vi "SUBVI_Image_to_Binary.vi"(11 "Image-in":T1) -> (0 "Red Binary":string[][](array[string]), 1 "Red Number":u8[][](array[numeric]), 2 "Blue Number":u8[][](array[numeric]), 3 "image_width":i32, 4 "Green Number":u8[][](array[numeric]), 5 "image_length":i32, 6 "Green Binary":string[][](array[string]), 7 "Blue Binary":string[][](array[string]))   [LabVIEW 2021]
uses:
  <vilib>/vision/Image Controls.llb/IMAQ Image.ctl
  <vilib>/vision/NI_Vision_Development_Module.lvlib
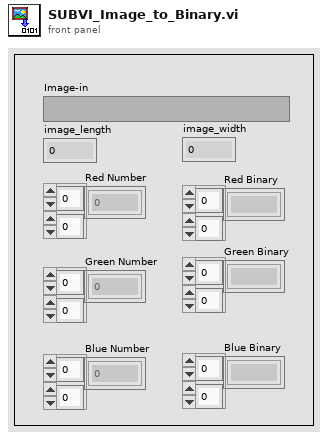
[diagram p1: front panel]
types:
  T1 = typedef "IMAQ Image.ctl" = refnum<image>
  T2 = cluster{"Red (or Hue) value":u8, "Green (or Sat) value":u8, "Blue (or Light or Val) value":u8}
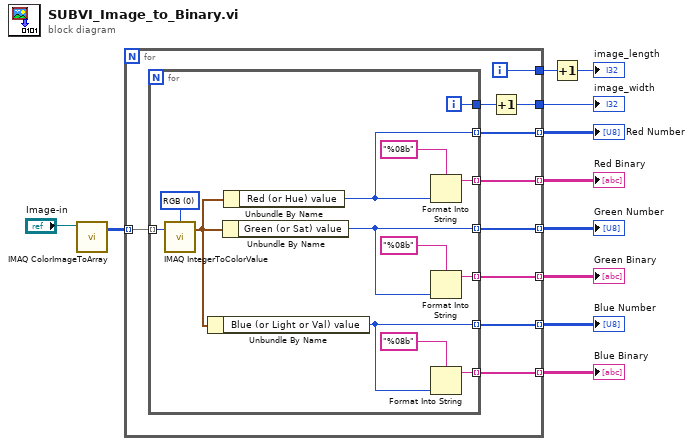
[diagram p0: block diagram]
diagram:
  n1 = call "IMAQ ColorImageToArray"("Image"="Image-in") -> ("Image Pixels (U32)"=w1:u32[][])  [unwired: 3 in, 2 out]
  n2 = for {
    tunnel: [w21] -> w4 mode=indexing
    tunnel: [w20] -> w3 mode=indexing
    tunnel: [w19] -> w5 mode=indexing
    tunnel: [w18] -> w7 mode=indexing
    tunnel: [w17] -> w6 mode=indexing
    tunnel: [w16] -> w2 mode=indexing
    tunnel: w1 -> [w15] mode=indexing
    tunnel: [w14] -> w8
    tunnel: [w12] -> w11
    i -> [w14]
    n3 = for {
      tunnel: [w28] -> w21 mode=indexing
      tunnel: [w29] -> w20 mode=indexing
      tunnel: [w31] -> w19 mode=indexing
      tunnel: [w27] -> w18 mode=indexing
      tunnel: [w26] -> w17 mode=indexing
      tunnel: [w25] -> w16 mode=indexing
      tunnel: w15 -> [w23] mode=indexing
      tunnel: [w22] -> w13
      i -> [w22]
      w24 = u16 0 items=["RGB", "HSL", "HSV", "HSI"] ("Color Mode")
      n4 = call "IMAQ IntegerToColorValue"("U32 value"=w23, "Color Mode"=w24) -> ("Color Value"=w34:T2)  [unwired: 3 in, 3 out]
      n5 = Unbundle By Name(w34) -> ("Blue (or Light or Val) value"=w31:u8)
      n6 = Unbundle By Name(w34) -> ("Green (or Sat) value"=w29:u8)
      n7 = Unbundle By Name(w34) -> ("Red (or Hue) value"=w28:u8)
      n8 = Format Into String(format string="%08b", w28) -> (resulting string=w27:string)  [unwired: 2 in, 1 out]
      n9 = Format Into String(format string="%08b", w29) -> (resulting string=w26:string)  [unwired: 2 in, 1 out]
      n10 = Format Into String(format string="%08b", w31) -> (resulting string=w25:string)  [unwired: 2 in, 1 out]
    }
    n11 = Increment(x=w13) -> (x+1=w12:i32)
  }
  "image_width" <- w11
  "Red Binary" <- w7
  "Green Binary" <- w6
  "Blue Number" <- w5
  "Red Number" <- w4
  "Green Number" <- w3
  "Blue Binary" <- w2
  n12 = Increment(x=w8) -> (x+1=→"image_length":i32)
